vi "readoutport.vi"() -> ()   [LabVIEW 2013]
panel:
  in  "Readout port":u32
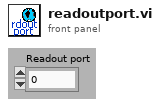
[diagram p1: front panel]
diagram:
